vi "Surpinski's Triangle.vi"() -> ()   [LabVIEW 2020]
uses:
  <vilib>/numeric/Random Number (Range) DBL.vi
  <vilib>/numeric/Random Number (Range) U64.vi
  <vilib>/numeric/sub_Random U32.vi
panel:
  out "Random Starting Point":cluster{"X":dbl, "Y":dbl}
  in  "Number of Points":i32
  in  "X":dbl[](array[numeric])
  in  "Y":dbl[](array[numeric])
  out "XY Graph":cluster{"X":dbl, "Y":dbl}[](graph)
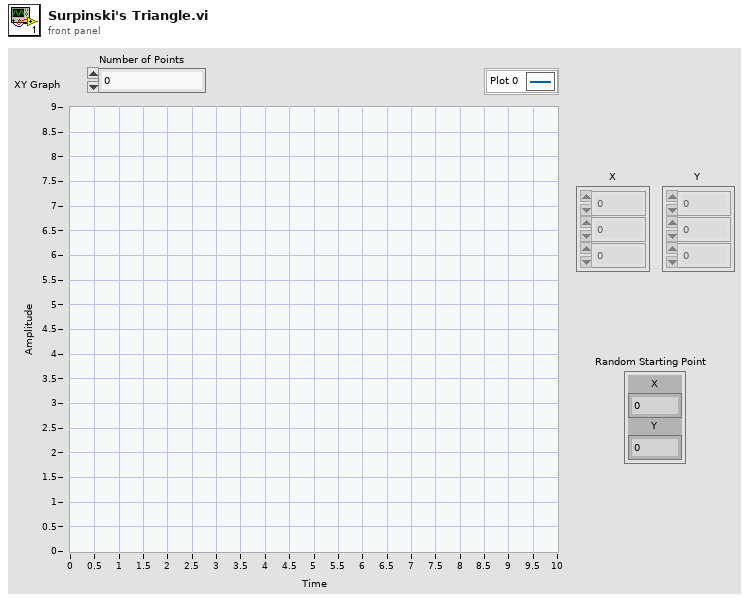
[diagram p1: front panel]
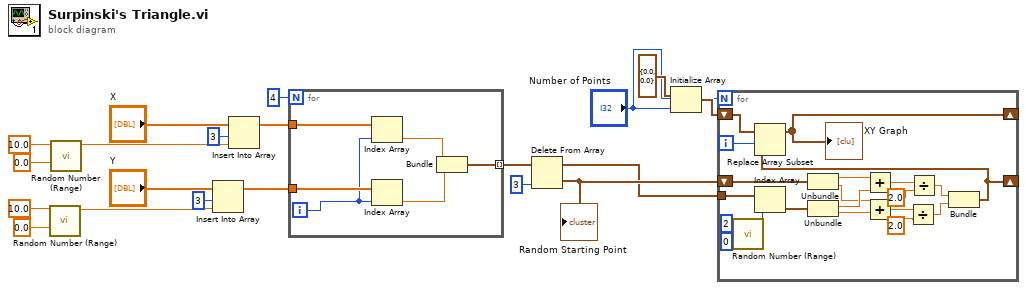
[diagram p0: block diagram]
diagram:
  n1 = call-poly <vilib>:"Random Number (Range).vi"("lower bound (0)"=0.0, "upper bound (100)"=10.0) -> ("number"=w12:dbl)  [unwired: 9 in]
  n2 = call-poly <vilib>:"Random Number (Range).vi"("lower bound (0)"=0.0, "upper bound (100)"=10.0) -> ("number"=w17:dbl)  [unwired: 9 in]
  n3 = Insert Into Array(array="Y", index=3, new element=w12) -> (w9:dbl[])
  n4 = Insert Into Array(array="X", index=3, new element=w17) -> (w10:dbl[])
  n5 = for {
    N: 4 -> [_]
    tunnel: w10 -> [w26]
    tunnel: w9 -> [w25]
    tunnel: [w21] -> w5 mode=indexing
    i -> [w22]
    n6 = Index Array(array=w26, index=w22) -> (element=w24:dbl)
    n7 = Index Array(array=w25, index=w22) -> (element=w23:dbl)
    n8 = Bundle("Numeric"=w24, "Numeric"=w23) -> (w21:cluster{"Numeric":dbl, "Numeric":dbl})  [unwired: 1 in]
  }
  n9 = Delete From Array(array=w5, index=3) -> (deleted portion=w3:cluster{"Numeric":dbl, "Numeric":dbl}, array with subset deleted=w2:cluster{"Numeric":dbl, "Numeric":dbl}[])  [unwired: 1 in]
  "Random Starting Point" <- w3
  n10 = Initialize Array(cluster{"Numeric":dbl, "Numeric":dbl} {"Numeric"=0.0, "Numeric"=0.0} ("output cluster"), "Number of Points") -> (w6:cluster{"Numeric":dbl, "Numeric":dbl}[])
  n11 = for {
    N: "Number of Points" -> [_]
    shift-right: [w27] -> _
    shift-left: w3 -> [w39]
    shift-right: [w44] -> _
    shift-left: w6 -> [w46]
    tunnel: w2 -> [w40]
    i -> [w45]
    n12 = call-poly <vilib>:"Random Number (Range).vi"("lower bound (0)"=u64 0, "upper bound (100)"=u64 2) -> ("number"=w41:u64)  [unwired: 9 in]
    n13 = Index Array(array=w40, index=w41) -> (element=w38:cluster{"Numeric":dbl, "Numeric":dbl})
    n14 = Unbundle(w39) -> ("Numeric"=w37:dbl, "Numeric"=w35:dbl)
    n15 = Unbundle(w38) -> ("Numeric"=w36:dbl, "Numeric"=w34:dbl)
    n16 = Add(x=w37, y=w36) -> (x+y=w32:dbl)
    n17 = Add(x=w35, y=w34) -> (x+y=w31:dbl)
    n18 = Divide(x=w31, y=2.0) -> (x/y=w28:dbl)
    n19 = Divide(x=w32, y=2.0) -> (x/y=w29:dbl)
    n20 = Bundle(w29, w28) -> (w27:cluster{dbl, dbl})  [unwired: 1 in]
    n21 = Replace Array Subset(array=w46, new element=w27, index=w45) -> (w44:cluster{"Numeric":dbl, "Numeric":dbl}[])
    "XY Graph" <- w44
  }
